vi "LINX - BlinkM Smart LED.vi"() -> ()   [LabVIEW 2011, in "LVH-LINX.lvlib"]
doc: "Set the color of a BlinkM Smart LED."
uses:
  vi.lib/LabVIEW Hacker/LINX/LVH-LINX.lvlib
  vi.lib/LabVIEW Hacker/LINX/Public/Sensors/BlinkM/BlinkM.lvlib
panel:
  out "Loop Rate (Hz)":u32
  in  "Serial Port":refnum<visa-resource-name>
  in  "Stop Button":bool
  out "LED Color":u32(colorbox)
  in  "Blue":u8(slide) scale=0.0..255.0
  in  "Green":u8(slide) scale=0.0..255.0
  in  "Red":u8(slide) scale=0.0..255.0
  # "Circuit Schematic"
  # "LINX Device Settings"
  # "BlinkM Color"
  # "BlinkM Smart LED Example\n\nThis example demonstrates how to set the color of a BlinkM smart LED and assumes\nthe BlinkM is connected to I2C channel 0 and is the only device on the bus.\n\nNote: This example is configured to use a serial interface but can easily be modified\nto use TCP or run on myRIO.\n\nInstructions\n1. Select the COM Port associated with the LINX Device.\n2. Click the Run Arrow.\n3. Adjust the Red Green and Blue sliders to change the BlinkM color."
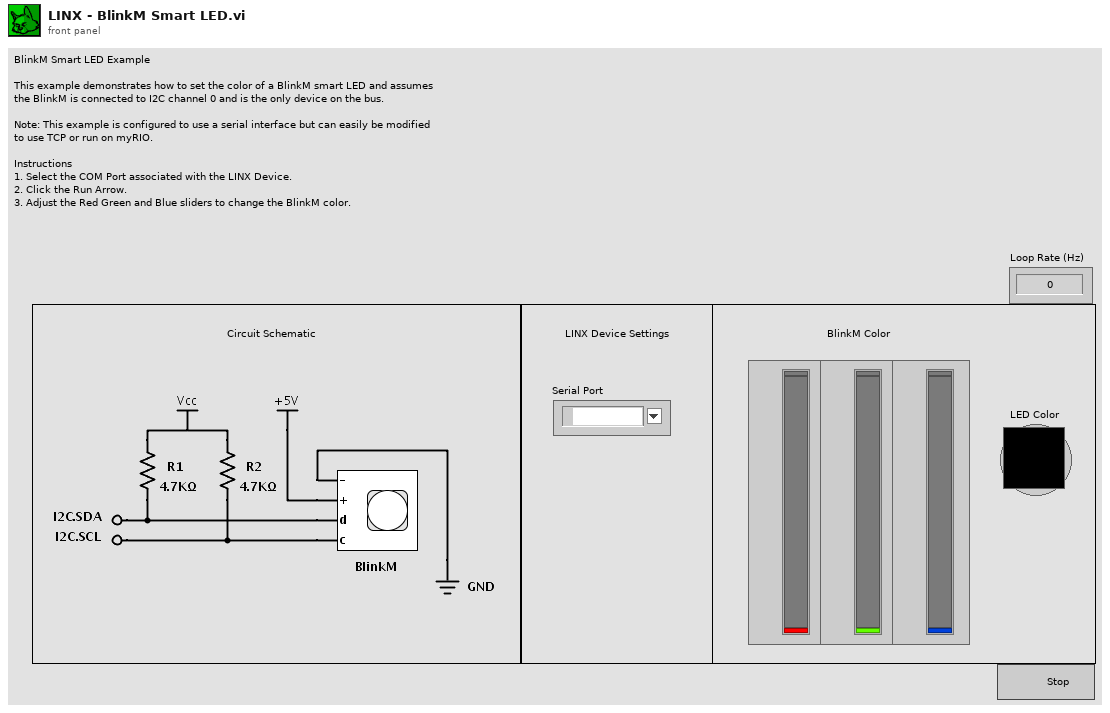
[diagram p1: front panel]
types:
  T1 = typedef "LVH-LINX.lvlib/LINX Ref.ctl" = cluster{"Platform":T2, "Interface":T3, "LINX Device Config":T4}
  T2 = typedef "LVH-LINX.lvlib/Platform.ctl" = enum16{"LINX", "myRIO"}
  T3 = typedef "LVH-LINX.lvlib/Interface.ctl" = enum16{"Serial", "TCP"}
  T4 = typedef "LVH-LINX.lvlib/Device.lvlib/LINX Device Config.ctl" = cluster{"Interface":T3, "COM Port":refnum<visa-resource-name>, "TCP Configuration":T5, "Device Family":T6, "Device ID":u8, "Device Name":string, "TCP Ref":refnum<k5>, "Channels":T7}
  T5 = typedef "LVH-LINX.lvlib/Device.lvlib/TCP Config.ctl" = cluster{"IP Address":string, "Port":u16}
  T6 = typedef "LVH-LINX.lvlib/Device Family.ctl" = enum8{"National Instruments", "Digilent", "Arduino"}
  T7 = typedef "LVH-LINX.lvlib/Channels.ctl" = cluster{"DI Channels":u8[], "DO Channels":u8[], "AI":u8[], "AO":u8[], "PWM":u8[], "QE":u8[], "UART":u8[], "I2C 2":u8[], "SPI":u8[], "CAN":u8[], "AI Ref (V)":dbl, "AO Resolution (Bits)":u8, "AO Ref (V)":dbl}
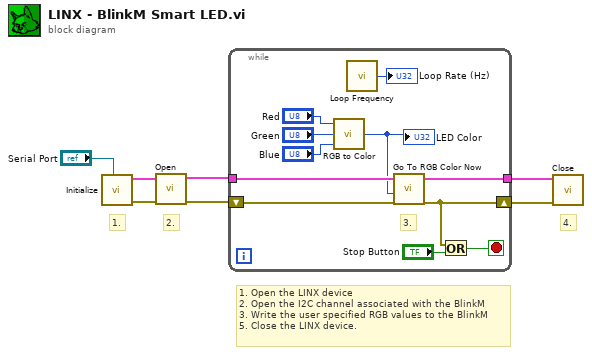
[diagram p0: block diagram]
diagram:
  # "4."
  # "2."
  # "1."
  # "1. Open the LINX device\n2. Open the I2C channel associated with the BlinkM\n3. Write the user specified RGB values to the BlinkM\n5. Close the LINX device."
  n1 = call "Initialize.vi"("Serial Port"="Serial Port") -> ("Error Out"=w3:errorcluster, "LINX Ref"=w4:T1)  [unwired: 8 in, 1 out]
  n2 = call "Open.vi"("Error In"=w3, "LINX Resource"=w4) -> ("Error Out"=w1:errorcluster, "LINX Resource"=w2:T1)  [unwired: 8 in]
  n3 = while {
    tunnel: w2 -> [w13]
    tunnel: [w12] -> w6
    shift-right: [w14] -> w7
    shift-left: w1 -> [w15]
    stop <- w18 stop-if-true
    # "3."
    n4 = call <vilib>:"RGB to Color.vi"("B"="Blue", "G"="Green", "R"="Red") -> ("Color"=w11:u32)
    "LED Color" <- w11
    n5 = call "Loop Frequency.vi"() -> ("Loop Rate (Hz)"=→"Loop Rate (Hz)":u32)
    n6 = call "Go To RGB Color Now.vi"("Error In"=w15, "Color"=w11, "LINX Resource"=w13) -> ("Error Out"=w14:errorcluster, "LINX Resource"=w12:T1)  [unwired: 7 in]
    n7 = Or(x=w14, y="Stop Button") -> (x .or. y?=w18:bool)
  }
  n8 = call "Close.vi"("Error In"=w7, "LINX Resource"=w6) -> ()  [unwired: 8 in, 2 out]
